vi "Get gRPC Method FullName.vi"(8 "error in (no error)":errorcluster, 11 "Method ref in":u64) -> (0 "error out":errorcluster, 2 "Method Full Name":string, 3 "Method ref out":u64)   [LabVIEW 2019, in "gRPC Template Creation Utility.lvlib"]
uses:
  gRPC Template Creation Utility.lvlib
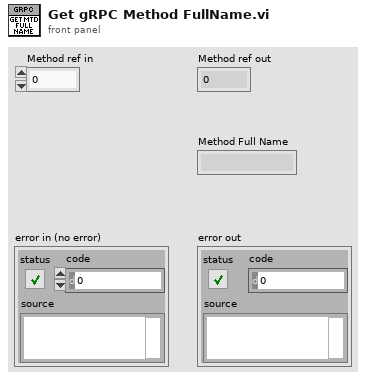
[diagram p1: front panel]
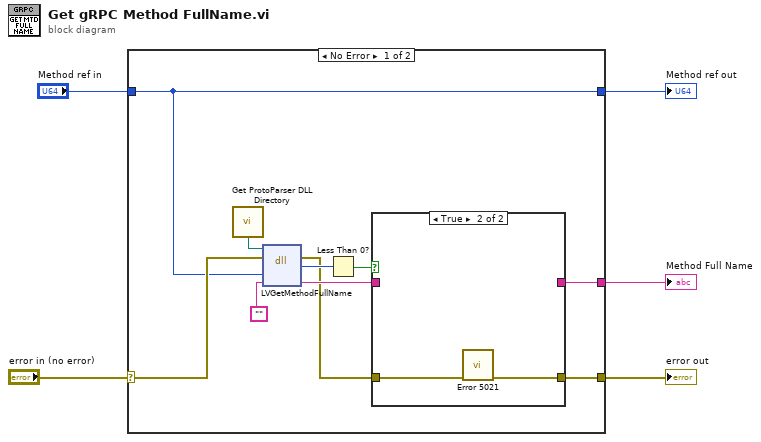
[diagram p0: block diagram]
diagram:
  n1 = case shown="No Error" "error in (no error)" {
    selector: "error in (no error)" -> [w14 w21]
    tunnel: "Method ref in" -> [w13 w20]
    tunnel: [w8 _] -> w4
    tunnel: [w13 w20] -> w2
    tunnel: [w7 w21] -> w1
    frame No Error {
      n2 = call "Get ProtoParser DLL Directory.vi"() -> ("Proto Parser Directory"=w12:path)
      n3 = dll-call lib="C:/Users/XEnderMD/Desktop/LV gRPC/labview source/gRPC Scripting Tools/Proto Parser API/dll/labview_grpc_generator.dll" fn="LVGetMethodFullName"(path in=w12, error in=w14, "method"=w13, "methodName"="") -> (error out=w6:errorcluster, "return type"=w11:i32, "methodName"=w9:string)  [unwired: 2 in, 1 out]
      n4 = Less Than 0?(x=w11) -> (x < 0?=w10:bool)
      n5 = case shown="True" w10 {
        tunnel: w9 -> [w17 _]
        tunnel: [w17 _] -> w8
        tunnel: [w16 w19] -> w7
        tunnel: w6 -> [w16 w18]
        frame False {
        }
        frame True {
          n6 = call "Error 5021.vi"("error in (no error)"=w18) -> ("error out"=w19:errorcluster)  [unwired: 10 in]
        }
      }
    }
    frame Error {
    }
  }
  "Method Full Name" <- w4
  "Method ref out" <- w2
  "error out" <- w1
